vi "GOMDBTS2048 spectral Is Enabled.vi"(8 "error in (no error)":errorcluster, 10 "enabled":bool, 11 "handle":i32) -> (0 "error out":errorcluster, 2 "enabled out":bool, 3 "function return":i32)   [LabVIEW 2015, in "GOMDBTS2048.lvlib"]
doc: "GOBTS2048DLL int __stdcall GOMDBTS2048_spectralIsEnabled(int handle, bool* enabled);"
uses:
  GOMDBTS2048.lvlib
  runtime/GOMDBTS2048.dll
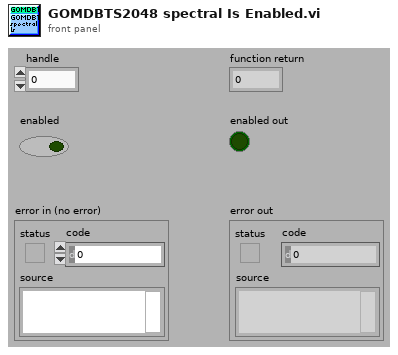
[diagram p1: front panel]
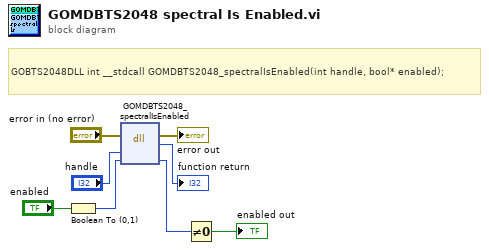
[diagram p0: block diagram]
diagram:
  # "GOBTS2048DLL int __stdcall GOMDBTS2048_spectralIsEnabled(int handle, bool* enabled);"
  n1 = Boolean To (0,1)(Boolean="enabled") -> (0, 1=w5:i16)
  n2 = dll-call lib="C:/Users/rkoch/Documents/GO_Library/runtime/GOMDBTS2048.*" fn="GOMDBTS2048_spectralIsEnabled"(error in="error in (no error)", "handle"="handle", "enabled"=w5) -> (error out=→"error out":errorcluster, →"function return":i32, "enabled"=w3:u8)  [unwired: 3 in, 1 out]
  n3 = Not Equal To 0?(x=w3) -> (x != 0?=→"enabled out":bool)
